vi "deleteTagfromTree.vi"(8 "error in (no error)":errorcluster, 9 "Delete Children?":bool, 10 "Tag":string, 11 "Tree Ref":refnum<vi>) -> (0 "error out":errorcluster, 3 "Tree ref out":refnum<vi>)   [LabVIEW 2010]
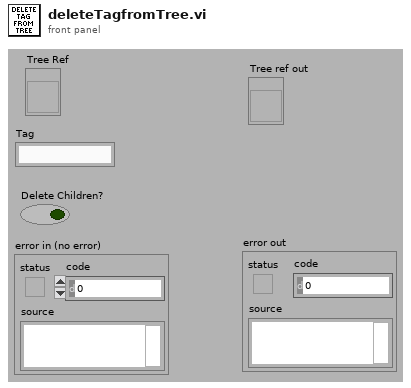
[diagram p1: front panel]
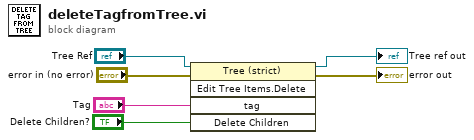
[diagram p0: block diagram]
diagram:
  n1 = invoke on="Invoke Node" class="Tree (strict)" method="Edit Tree Items.Delete"(reference="Tree Ref", error in="error in (no error)", "tag"="Tag", "Delete Children"="Delete Children?") -> (reference out=→"Tree ref out":refnum<vi>, error out=→"error out":errorcluster)  [unwired: 1 in, 3 out]
